vi "curv test.vi"() -> ()   [LabVIEW 2019]
panel:
  in  "sensor thr array":dbl[](array[numeric])
  in  "counting role 2":T1(ring)
  in  "curv sw info":dbl[](array[numeric])
  out "Col5 CURV(mm)":dbl format="%#_2g"
  out "Overal CURV(mm)":dbl format="%#_2g"
  out "CURV (mm)":dbl format="%#_3g"
  out "curv sit":bool
  out "SWL 2":bool
  out "SWR 2":bool
  out "Col4 CURV(mm)":dbl format="%#_2g"
  out "Col3 CURV(mm)":dbl format="%#_2g"
  out "Col2 CURV(mm)":dbl format="%#_2g"
  out "Col1 CURV(mm)":dbl format="%#_2g"
  out "SideWall Sensors Graph":dynamicdata(graph)
  out "Curvness Sensors Graph":dynamicdata(graph)
  out "stop ok":bool caption="OK"
  out "Col. Count":bool
  out "Col\n NUM":dbl format="%#.1g"
  out "avg data array":dbl[](array[numeric])
  out "capture triger":bool
  out "Plt Count":bool
  out "Speed :":string="178"
  out "capture or not?":bool=TRUE
  in  "capture":bool
  out "sensor error in":errorcluster
  out "sensor errors":errorcluster
  out "counting role":T1(ring)
  out "ch sw sensor2":dbl
  out "ch sw sensor1":dbl
  out "ch sensor3":dbl
  out "ch sensor2":dbl
  out "ch sensor1":dbl
  out "3rd sensor thr":u16=30000
  out "2nd sensor thr":u16=30000
  out "1st sensor thr":u32=26500
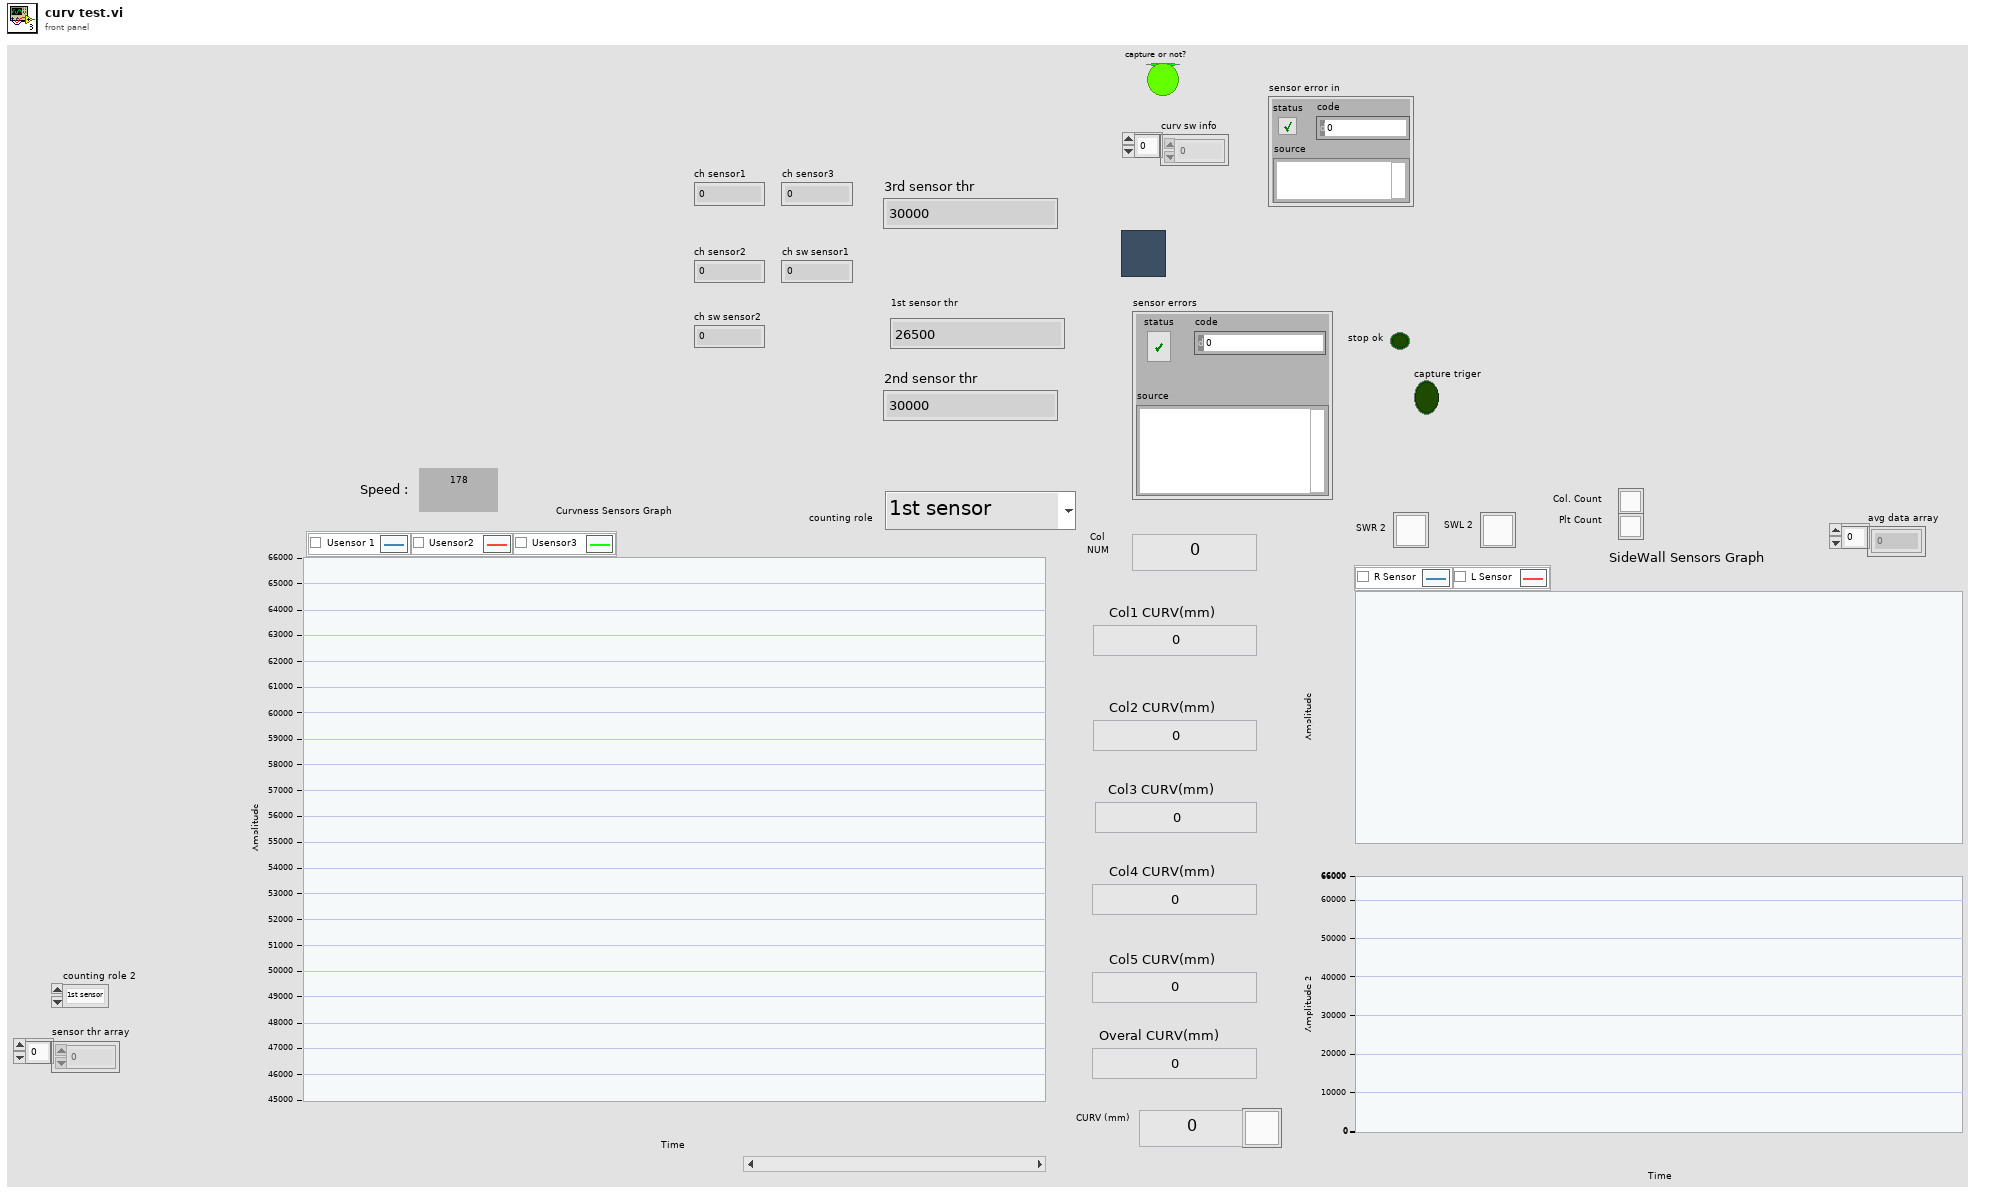
[diagram p1: front panel]
types:
  T1 = enum16{"1st sensor", "2nd sensor", "3rd sensor", "1st+2nd", "1st+3rd", "2nd+3rd", "1st+2nd+3rd"}
  T2 = cluster{"ch sensor1":dbl, "ch sensor2":dbl, "ch sensor3":dbl, "ch sw sensor1":dbl, "ch sw sensor2":dbl}
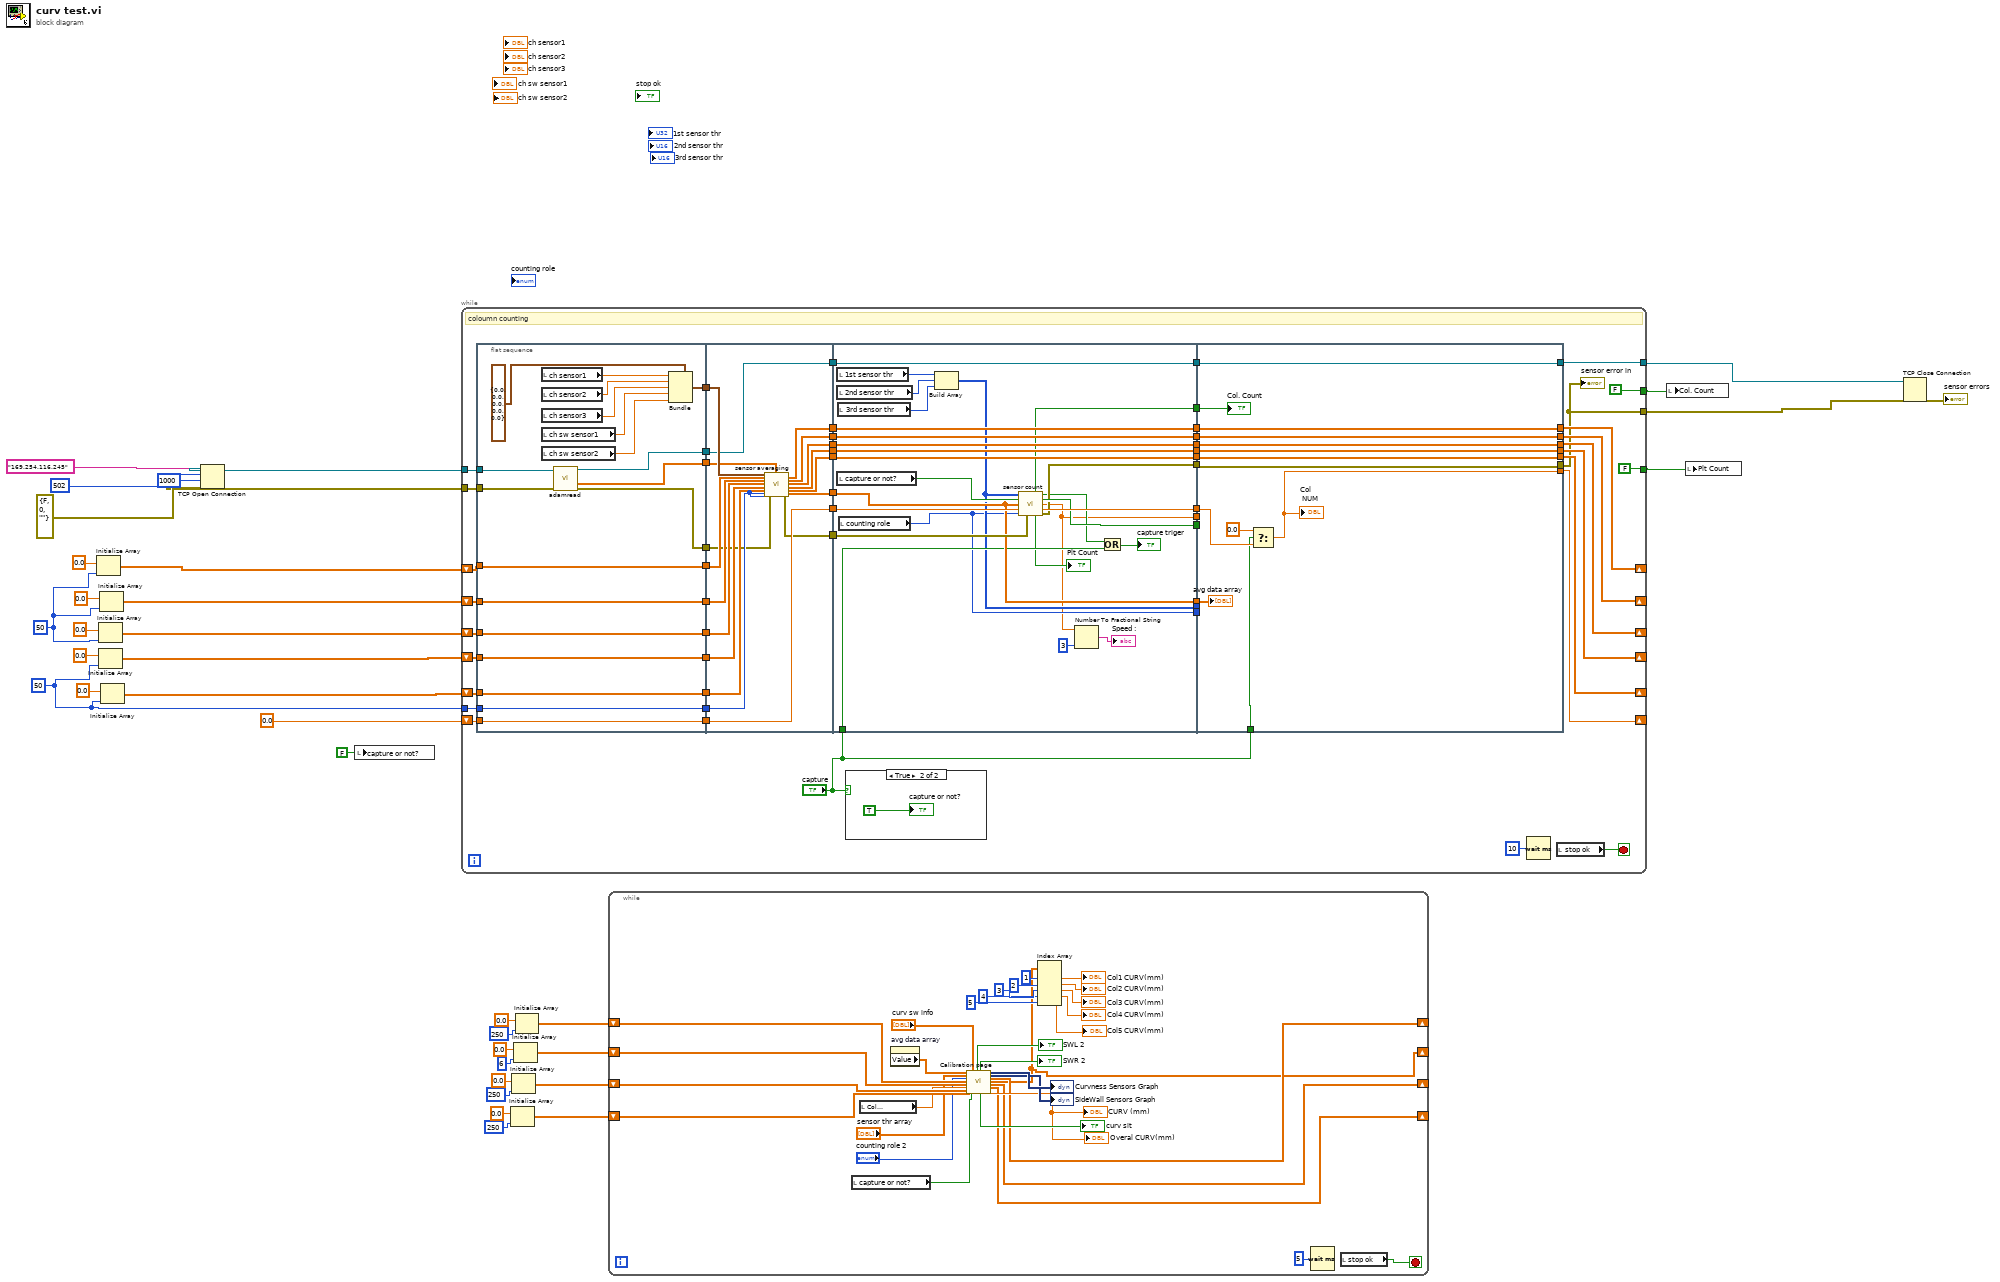
[diagram p0: block diagram]
diagram:
  w22 = 50 ("dimension size")
  w31 = 50 ("dimension size")
  n1 = Initialize Array(0.0 ("element"), w31) -> (w27:dbl[])
  n2 = Initialize Array(0.0 ("element"), w31) -> (w25:dbl[])
  n3 = Initialize Array(0.0 ("element"), w22) -> (w24:dbl[])
  n4 = Initialize Array(0.0 ("element"), w31) -> (w26:dbl[])
  n5 = Initialize Array(0.0 ("element"), w22) -> (w23:dbl[])
  n6 = TCP Open Connection(address="169.254.116.245" ("IP #"), remote port or service name=u16 502 ("Remote Port"), timeout ms (60000)=1000, error in (no error)=errorcluster {"status"=FALSE, "code"=0, "source"=""}) -> (connection ID=w35:refnum<k5>, error out=w34:errorcluster)  [unwired: 1 in]
  n7 = local write "capture or not?"(FALSE ("capture or not?")) -> ()
  n8 = while {
    tunnel: w35 -> [w92]
    tunnel: w34 -> [w91]
    shift-right: [w73] -> _
    shift-left: w27 -> [w89]
    shift-right: [w68] -> _
    shift-left: w26 -> [w86]
    shift-right: [w67] -> _
    shift-left: w25 -> [w84]
    shift-right: [w66] -> _
    shift-left: w24 -> [w82]
    shift-right: [w65] -> _
    shift-left: w23 -> [w80]
    tunnel: w22 -> [w78]
    shift-right: [w50] -> _
    shift-left: 0.0 ("element") -> [w64]
    tunnel: [w49] -> w20
    tunnel: [w45] -> w19
    tunnel: [FALSE ("Col. Count")] -> w15
    tunnel: [FALSE ("Plt Count")] -> w14
    stop <- w93 stop-if-true
    # "coloumn counting"
    n9 = flat-sequence {
      tunnel: w92 -> [w113]
      tunnel: w91 -> [w112]
      tunnel: [w105] -> w90
      tunnel: w89 -> [w104]
      tunnel: [w104] -> w88
      tunnel: [w103] -> w87
      tunnel: w86 -> [w103]
      tunnel: [w102] -> w85
      tunnel: w84 -> [w102]
      tunnel: [w101] -> w83
      tunnel: w82 -> [w101]
      tunnel: [w100] -> w81
      tunnel: w80 -> [w100]
      tunnel: [w99] -> w79
      tunnel: w78 -> [w99]
      tunnel: [w98] -> w77
      tunnel: [w97] -> w76
      tunnel: w64 -> [w96]
      tunnel: [w96] -> w62
      tunnel: [w95] -> w46
      tunnel: w90 -> [w131]
      tunnel: w88 -> [w130]
      tunnel: w87 -> [w129]
      tunnel: w85 -> [w128]
      tunnel: w83 -> [w127]
      tunnel: w81 -> [w126]
      tunnel: w79 -> [w125]
      tunnel: w77 -> [w124]
      tunnel: w76 -> [w123]
      tunnel: [w122] -> w75
      tunnel: [w121] -> w74
      tunnel: [w120] -> w72
      tunnel: [w119] -> w71
      tunnel: [w118] -> w70
      tunnel: [w117] -> w69
      tunnel: [w116] -> w63
      tunnel: w62 -> [w116]
      tunnel: [w115] -> w61
      tunnel: [w114] -> w47
      tunnel: w46 -> [w114]
      tunnel: w75 -> [w146]
      tunnel: w74 -> [w154]
      tunnel: w72 -> [w153]
      tunnel: w71 -> [w152]
      tunnel: w70 -> [w151]
      tunnel: w69 -> [w150]
      tunnel: w63 -> [w148]
      tunnel: w61 -> [w147]
      tunnel: [w154] -> w60
      tunnel: [w153] -> w59
      tunnel: [w152] -> w58
      tunnel: [w151] -> w57
      tunnel: [w150] -> w56
      tunnel: [w146] -> w55
      tunnel: [w145] -> w54
      tunnel: [w134] -> w53
      tunnel: [w144] -> w52
      tunnel: [w143] -> w51
      tunnel: [w142] -> w48
      tunnel: w47 -> [w142]
      tunnel: [w141] -> w43
      tunnel: "capture" -> [w139]
      tunnel: [w137] -> w39
      tunnel: [w136] -> w38
      tunnel: [w166] -> w65
      tunnel: [w167] -> w66
      tunnel: [w168] -> w67
      tunnel: [w169] -> w68
      tunnel: [w170] -> w73
      tunnel: [w159] -> w50
      tunnel: [w161] -> w49
      tunnel: [w163] -> w45
      tunnel: w43 -> [w160]
      tunnel: w48 -> [w163]
      tunnel: "capture" -> [w162]
      tunnel: w51 -> [w161]
      tunnel: w52 -> [_]
      tunnel: w53 -> [_]
      tunnel: w54 -> [w164]
      tunnel: w55 -> [w158]
      tunnel: w56 -> [w166]
      tunnel: w57 -> [w167]
      tunnel: w58 -> [w168]
      tunnel: w59 -> [w169]
      tunnel: w60 -> [w170]
      tunnel: w39 -> [_]
      tunnel: w38 -> [_]
      frame #0 {
        n10 = local read "ch sensor1"() -> (w106:dbl)
        n11 = local read "ch sensor2"() -> (w107:dbl)
        n12 = local read "ch sensor3"() -> (w108:dbl)
        n13 = local read "ch sw sensor1"() -> (w109:dbl)
        n14 = local read "ch sw sensor2"() -> (w110:dbl)
        n15 = call "adamread.vi"("TCP Connection Refnum in"=w113, "error in (no error)"=w112) -> ("TCP Connection Refnum (dup)"=w95:refnum<k5>, "Slave Input Registers 2"=w98:dbl[], "error out 2"=w97:errorcluster)  [unwired: 11 in]
        n16 = Bundle(cluster=T2 {"ch sensor1"=0.0, "ch sensor2"=0.0, "ch sensor3"=0.0, "ch sw sensor1"=0.0, "ch sw sensor2"=0.0}, "ch sensor1"=w106, "ch sensor2"=w107, "ch sensor3"=w108, "ch sw sensor1"=w109, "ch sw sensor2"=w110) -> (w105:T2)
      }
      frame #1 {
        n17 = call "sensor averaging.vi"("sensor chanel cluster"=w131, "array"=w130, "array 2"=w129, "array 3"=w128, "array 4"=w127, "array 5"=w126, "avg win1"=w125, "avg win2"=w125, "array sensor in"=w124, "error in"=w123) -> ("error out"=w115:errorcluster, "output array"=w121:dbl[], "output array 2"=w120:dbl[], "output array 3"=w119:dbl[], "output array 4"=w118:dbl[], "output array 5"=w117:dbl[], "avg data array"=w122:dbl[])  [unwired: 10 in, 1 out]
      }
      frame #2 {
        n18 = local read "1st sensor thr"() -> (w155:u32)
        n19 = local read "2nd sensor thr"() -> (w156:u16)
        n20 = local read "capture or not?"() -> (w149:bool)
        n21 = local read "3rd sensor thr"() -> (w157:u16)
        n22 = local read "counting role"() -> (w136:T1)
        n23 = Build Array(w155, w156, w157) -> (w137:u32[])
        n24 = call "sensor count.vi"("sensor thr array"=w137, "capture y or no ?"=w149, "sensor data"=w146, "counter input"=w148, "counting role"=w136, "error in"=w147) -> ("column count"=w141:bool, "capture trigger"=w140:bool, "sensor counter"=w144:bool, "speed"=w134:dbl, "counter out"=w145:dbl, "pallet detect"=→"Plt Count":bool, "error out"=w143:errorcluster)  [unwired: 3 in]
        n25 = Number To Fractional String(number=w134, precision (6)=i16 3) -> (F-format string=→"Speed :":string)  [unwired: 2 in]
        n26 = Or(x=w140, y=w139) -> (x .or. y?=→"capture triger":bool)
      }
      frame #3 {
        n27 = Select(t=0.0, s=w162, f=w164) -> (s? t:f=w159:dbl)
        "Col\n NUM" <- w159
        "Col. Count" <- w160
        "avg data array" <- w158
      }
    }
    n28 = case shown="True" "capture" {
      frame False {
      }
      frame True {
        "capture or not?" <- TRUE ("Boolean")
      }
    }
    n29 = Wait (ms)(milliseconds to wait=u32 10) -> ()  [unwired: 1 out]
    n30 = local read "stop ok"() -> (w93:bool)
    "sensor error in" <- w49
  }
  n31 = Initialize Array(0.0 ("element"), 250 ("dimension size")) -> (w2:dbl[])
  n32 = Initialize Array(0.0 ("element"), 250 ("dimension size")) -> (w3:dbl[])
  n33 = Initialize Array(0.0 ("element"), 6 ("dimension size")) -> (w4:dbl[])
  n34 = Initialize Array(0.0 ("element"), 250 ("dimension size")) -> (w5:dbl[])
  n35 = while {
    shift-right: [w177] -> _
    shift-left: w5 -> [w186]
    shift-right: [w171] -> _
    shift-left: w4 -> [w185]
    shift-right: [w176] -> _
    shift-left: w3 -> [w184]
    shift-right: [w175] -> _
    shift-left: w2 -> [w183]
    stop <- w172 stop-if-true
    n36 = local read "capture or not?"() -> (w174:bool)
    n37 = local read "Col\n NUM"() -> (w182:dbl)
    n38 = property on="avg data array" class="Arr (strict)"() -> ("Value"=w181:dbl[])  [unwired: 2 in, 2 out]
    n39 = call "Calibration page.vi"("sensor data array"=w181, "sensor thr array"="sensor thr array", "counting role"="counting role 2", "sensor1 array"=w186, "curv array in"=w185, "count in"=w182, "sensor2 array"=w184, "sensor3 array"=w183, "curv sw info"="curv sw info", "capture"=w174) -> ("Left Sidewall"=→"SWL 2":bool, "Right Sidewall"=→"SWR 2":bool, "curv sit"=→"curv sit":bool, "Curvness Sensors Graph"=→"Curvness Sensors Graph":dynamicdata, "SideWall Sensors Graph"=→"SideWall Sensors Graph":dynamicdata, "sensor1 array out"=w177:dbl[], "curv array out"=w171:dbl[], "sensor2 array out"=w176:dbl[], "sensor3 array out"=w175:dbl[], "Pallet CURV (mm)"=→"CURV (mm)" →"Overal CURV(mm)":dbl)  [unwired: 7 in, 1 out]
    n40 = Index Array(array=w171, index #1=1 ("index"), index #2=2 ("index"), index #3=3 ("index"), index #4=4 ("index"), index #5=5 ("index")) -> (element #1=→"Col1 CURV(mm)":dbl, element #2=→"Col2 CURV(mm)":dbl, element #3=→"Col3 CURV(mm)":dbl, element #4=→"Col4 CURV(mm)":dbl, element #5=→"Col5 CURV(mm)":dbl)
    n41 = Wait (ms)(milliseconds to wait=u32 5) -> ()  [unwired: 1 out]
    n42 = local read "stop ok"() -> (w172:bool)
  }
  n43 = local write "Col. Count"(w15) -> ()
  n44 = local write "Plt Count"(w14) -> ()
  n45 = TCP Close Connection(connection ID=w19, error in (no error)=w20) -> (error out=→"sensor errors":errorcluster)  [unwired: 1 in, 1 out]
